vi "OAT Tachless Cursor Sorting.vi"(1 "Numeric":dbl format="%.2f", 2 "Array":T1(array[cluster]) {"Location"."Y" format="%.2f"; "Location"."X" format="%.2f"}) -> (0 "Array 2":T1(array[cluster]) {"Location"."Y" format="%.2f"; "Location"."X" format="%.2f"})   [LabVIEW 2017, in "SoundVib_Tachless.lvlib"]
uses:
  <vilib>/addons/Sound and Vibration/Order Analysis/Tachless/SoundVib_Tachless.lvlib
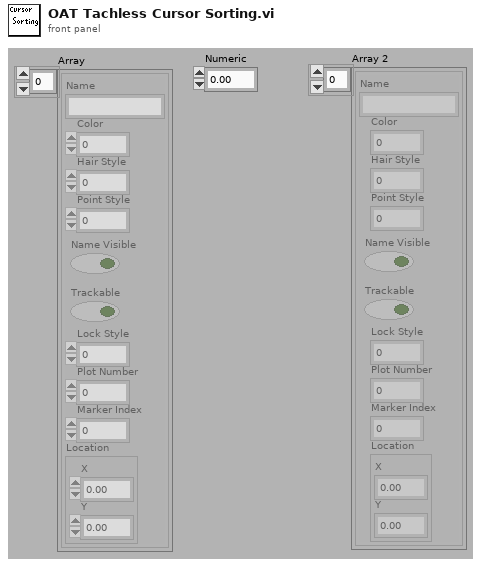
[diagram p1: front panel]
types:
  T1 = cluster{"Name":string, "Color":u32, "Hair Style":u8, "Point Style":u8, "Name Visible":bool, "Trackable":bool, "Lock Style":u32, "Plot Number":u32, "Marker Index":i32, "Location":cluster{"X":dbl, "Y":dbl}}[]
  T2 = cluster{"Name":string, "Color":u32, "Hair Style":u8, "Point Style":u8, "Name Visible":bool, "Trackable":bool, "Lock Style":u32, "Plot Number":u32, "Marker Index":i32, "Location":cluster{"X":dbl, "Y":dbl}}
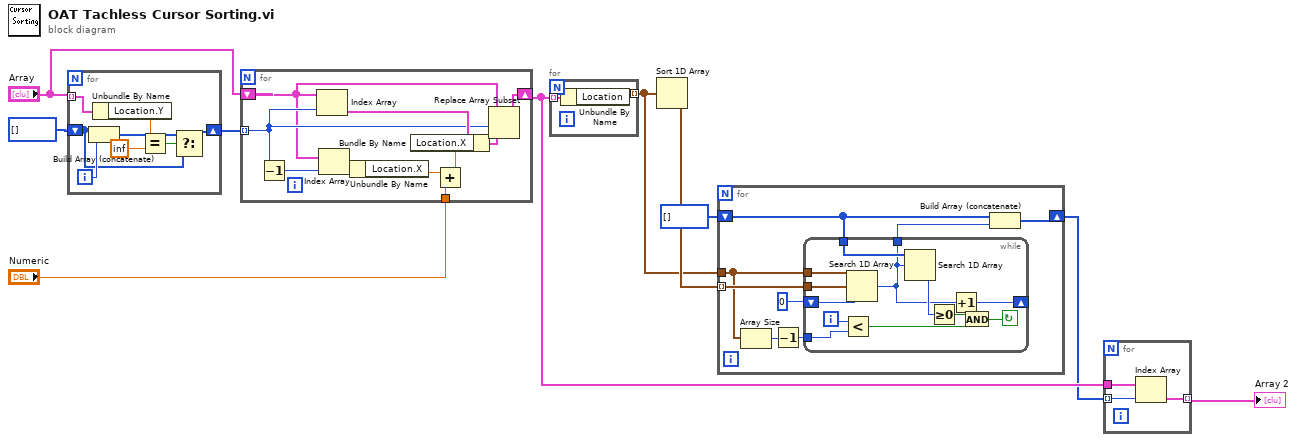
[diagram p0: block diagram]
diagram:
  n1 = for {
    tunnel: "Array" -> [w18] mode=indexing
    shift-right: [w11] -> w2
    shift-left: i32[] [] -> [w12]
    i -> [w14]
    n2 = Build Array (concatenate)(w12, w14) -> (w13:i32[])
    n3 = Unbundle By Name(w18) -> ("Location.Y"=w17:dbl)
    n4 = Equal?(x=w17, y=inf) -> (x = y?=w15:bool)
    n5 = Select(t=w13, s=w15, f=w12) -> (s? t:f=w11:i32[])
  }
  n6 = for {
    shift-right: [w19] -> w8
    shift-left: "Array" -> [w20]
    tunnel: w2 -> [w21] mode=indexing
    tunnel: "Numeric" -> [w24]
    n7 = Decrement(x=w21) -> (x-1=w27:i32)
    n8 = Index Array(array=w20, index=w21) -> (element=w28:T2)
    n9 = Index Array(array=w20, index=w27) -> (element=w26:T2)
    n10 = Unbundle By Name(w26) -> ("Location.X"=w25:dbl)
    n11 = Add(x=w25, y=w24) -> (x+y=w23:dbl)
    n12 = Bundle By Name(cluster=w28, "Location.X"=w23) -> (w22:T2)
    n13 = Replace Array Subset(array=w20, new element=w22, index=w21) -> (w19:T1)
  }
  n14 = for {
    tunnel: w8 -> [w30] mode=indexing
    tunnel: [w29] -> w9 mode=indexing
    n15 = Unbundle By Name(w30) -> ("Location"=w29:cluster{"X":dbl, "Y":dbl})
  }
  n16 = Sort 1D Array(array=w9) -> (sorted array=w10:cluster{"X":dbl, "Y":dbl}[])
  n17 = for {
    tunnel: w10 -> [w38] mode=indexing
    tunnel: w9 -> [w34]
    shift-right: [w37] -> w5
    shift-left: i32[] [] -> [w36]
    n18 = Array Size(array=w34) -> (size(s)=w33:i32)
    n19 = Decrement(x=w33) -> (x-1=w32:i32)
    n20 = while {
      tunnel: [w40] -> w31
      tunnel: w32 -> [w44]
      shift-left: 0 -> [w41]
      shift-right: [w39] -> _
      tunnel: w36 -> [w48]
      tunnel: w38 -> [w49]
      tunnel: w34 -> [w50]
      i -> [w45]
      stop <- w42 continue-if-true
      n21 = Less?(x=w45, y=w44) -> (x < y?=w43:bool)
      n22 = Search 1D Array(1D array=w50, element=w49, start index (0)=w41) -> (index of element=w40:i32)
      n23 = Search 1D Array(1D array=w48, element=w40) -> (index of element=w47:i32)  [unwired: 1 in]
      n24 = Greater Or Equal To 0?(x=w47) -> (x >= 0?=w46:bool)
      n25 = Increment(x=w40) -> (x+1=w39:i32)
      n26 = And(x=w46, y=w43) -> (x .and. y?=w42:bool)
    }
    n27 = Build Array (concatenate)(w36, w31) -> (w37:i32[])
  }
  n28 = for {
    tunnel: w8 -> [w53]
    tunnel: w5 -> [w52] mode=indexing
    tunnel: [w51] -> w6 mode=indexing
    n29 = Index Array(array=w53, index=w52) -> (element=w51:T2)
  }
  "Array 2" <- w6
